vi "Timeout.vi"(8 "error in (no error)":errorcluster, 10 "Data":variant, 11 "Thermocouples in":refnum<class "Thermocouples.lvclass">) -> (0 "error out":errorcluster, 3 "Thermocouples out":refnum<class "Thermocouples.lvclass">)   [LabVIEW 2015, in "AMS UI.lvlib" / "Thermocouples.lvclass"]
uses:
  Thermocouples.lvclass
  Thermocouples.lvclass/Thermocouples.ctl
  AMS Gas Actor/AMS Gas Actor.lvclass
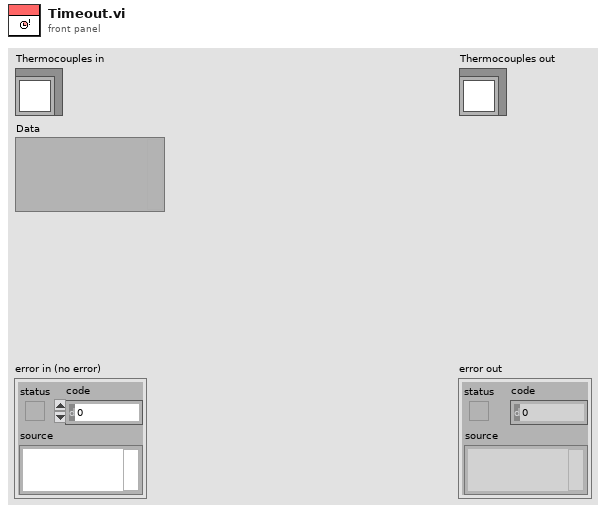
[diagram p1: front panel]
types:
  T1 = cluster{"Double":dbl, "Double":dbl, "Double":dbl, "Double":dbl, "Double":dbl, "Double":dbl}
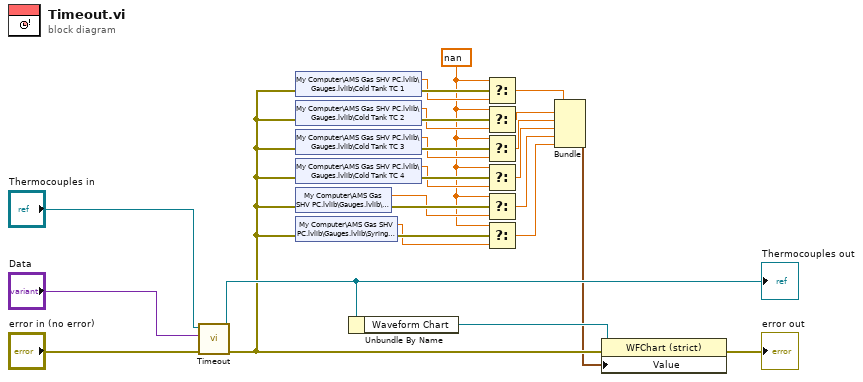
[diagram p0: block diagram]
diagram:
  w13 = nan ("t")
  n1 = call-parent "Timeout.vi"("error in (no error)"="error in (no error)", "Data"="Data", "eActor in"="Thermocouples in") -> ("error out"=w11:errorcluster, "eActor out"=w12:refnum<class "Thermocouples.lvclass">)  [unwired: 7 in]
  "Thermocouples out" <- w12
  n2 = shared-variable "My Computer\\AMS Gas SHV PC.lvlib\\Gauges.lvlib\\Cold Tank TC 1"(error in=w11) -> (w19:dbl, error out=w25:errorcluster)
  n3 = shared-variable "My Computer\\AMS Gas SHV PC.lvlib\\Gauges.lvlib\\Cold Tank TC 2"(error in=w11) -> (w18:dbl, error out=w23:errorcluster)
  n4 = shared-variable "My Computer\\AMS Gas SHV PC.lvlib\\Gauges.lvlib\\Cold Tank TC 3"(error in=w11) -> (w17:dbl, error out=w22:errorcluster)
  n5 = shared-variable "My Computer\\AMS Gas SHV PC.lvlib\\Gauges.lvlib\\Cold Tank TC 4"(error in=w11) -> (w16:dbl, error out=w21:errorcluster)
  n6 = shared-variable "My Computer\\AMS Gas SHV PC.lvlib\\Gauges.lvlib\\Piston TC"(error in=w11) -> (w15:dbl, error out=w20:errorcluster)
  n7 = shared-variable "My Computer\\AMS Gas SHV PC.lvlib\\Gauges.lvlib\\Syringe TC"(error in=w11) -> (w14:dbl, error out=w24:errorcluster)
  n8 = Unbundle By Name(w12) -> ("Waveform Chart"=w9:refnum<vi>)
  n9 = Select(t=w13, s=w25, f=w19) -> (s? t:f=w8:dbl)
  n10 = Select(t=w13, s=w23, f=w18) -> (s? t:f=w7:dbl)
  n11 = Select(t=w13, s=w22, f=w17) -> (s? t:f=w6:dbl)
  n12 = Select(t=w13, s=w21, f=w16) -> (s? t:f=w5:dbl)
  n13 = Select(t=w13, s=w20, f=w15) -> (s? t:f=w4:dbl)
  n14 = Select(t=w13, s=w24, f=w14) -> (s? t:f=w3:dbl)
  n15 = Bundle("Double"=w8, "Double"=w7, "Double"=w6, "Double"=w5, "Double"=w4, "Double"=w3) -> (w2:T1)  [unwired: 1 in]
  n16 = property class="WFChart (strict)"(reference=w9, error in=w11, "Value"=w2) -> (error out=→"error out":errorcluster)  [unwired: 1 out]
